vi "Read File.vi"(8 "error in (no error)":errorcluster, 10 "Path in":path, 11 "File Interface in":refnum<class "File Interface.lvclass">) -> (0 "error out":errorcluster, 2 "SysDef":T1 {"Tree"."Properties"."Type" items=["K_STRING", "K_BOOL", "K_I32", "K_U32", "K_DOUBLE", "K_U64", "K_VARIANT", "K_DEPENDENTFILE", "K_DEPENDENTNODE", "K_DATASOURCENODE", "K_U16", "K_DBLARR", "K_U32ARR", "K_I32ARR", "K_STRINGARR", "K_DICTIONARY", "K_DICTIONARYARR"]})   [LabVIEW 2018, in "ImportExport.lvlib" / "File Interface.lvclass"]
uses:
  Switch Configuration.llb/File Interface.lvclass
  Switch Configuration.llb/Advanced System Definition.lvlib
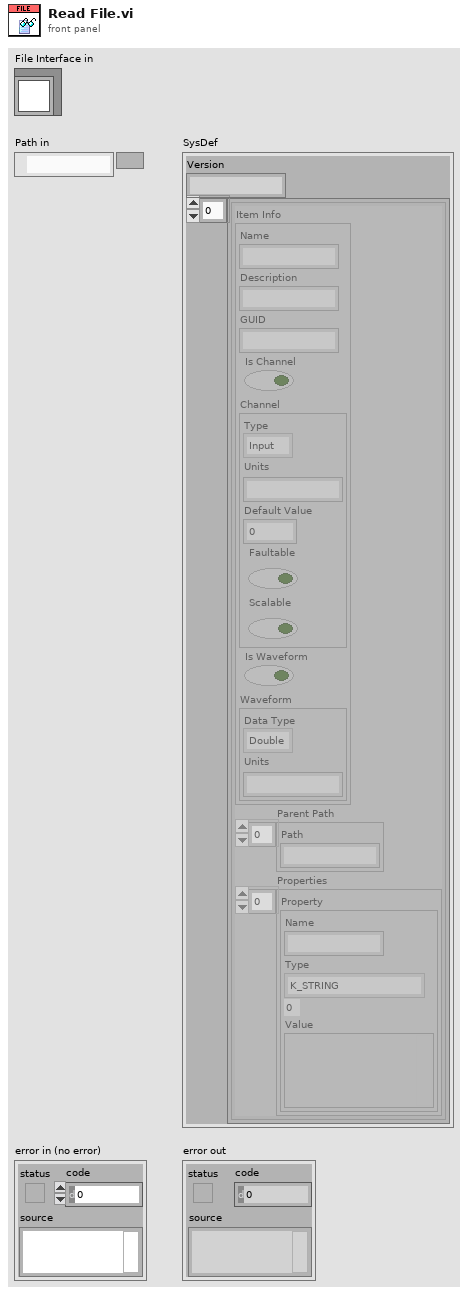
[diagram p1: front panel]
types:
  T1 = cluster{"Version":string, "Tree":cluster{"Item Info":cluster{"Name":string, "Description":string, "GUID":string, "Is Channel":bool, "Channel":cluster{"Type":enum16{"Input", "Output"}, "Units":string, "Default Value":dbl, "Faultable":bool, "Scalable":bool}, "Is Waveform":bool, "Waveform":cluster{"Data Type":enum16{"Double", "Complex Double"}, "Units":string}}, "Parent Path":string[], "Properties":cluster{"Name":string, "Type":i32, "Value":variant}[]}[]}
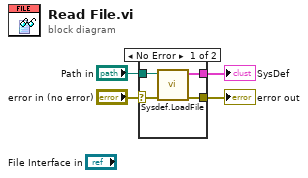
[diagram p0: block diagram]
diagram:
  n1 = case shown="No Error" "error in (no error)" {
    selector: "error in (no error)" -> [w6 w9]
    tunnel: [w5 w9] -> w3
    tunnel: "Path in" -> [w8 _]
    tunnel: [w7 _] -> w1
    frame No Error {
      n2 = call "Sysdef.LoadFile.vi"("error in (no error)"=w6, "Path in"=w8) -> ("error out"=w5:errorcluster, "SysDef"=w7:T1)  [unwired: 8 in]
    }
    frame Error {
    }
  }
  "error out" <- w3
  "SysDef" <- w1
